vi "Vision Research Phantom Series PhInt PhInterpolateColorPAR.vi"(0 "Camera Number (1)":u32=1, 2 "CFA":T2 {"CFA" items=["CFA_NONE", "CFA_VRI", "CFA_VRIV6", "CFA_BAYER", "CFA_BAYERFLIP"]}, 3 "Algorithm":T1=1 items=["FAST_ALGORITHM"=1, "BEST_ALGORITHM"=5, "NO_DEMOSAICING"=6], 4 "pPixel In":u8[](array[numeric]), 5 "Error In (no error)":errorcluster, 7 "BITMAPINFOHEADER":T3) -> (14 "Camera Number out":u32=1, 16 "pPixel Out":u8[](array[numeric]), 19 "Error Out":errorcluster)   [LabVIEW 2013, in "VRI.lvlib"]
doc: "PhInt.dll\n\nPhInterpolateColorPAR\nPhInterpolateColorPAR(int Width, int Height, int BitCount, unsigned char * pPixel, int CFA, int Algorithm );\n\nParameters Description\nWidth Image width\nHeight Image height\nBitCount Bits per pixel\npPixel Pixel array pointer\nAlgorithm Interpolation algorithm code (BEST_ALGOTITHM, FAST_ALGORITHM)\nReturn Void\nComments A replacement for LabView of the PhMakeColor function\n\nWritten by:\nBLOOMY CONTROLS, INC\nWINDSOR, CT 06095, USA\n860-298-9925\nwww.bloomy.com\nV1.0.0\nMay, 2004"
uses:
  VRI.lvlib
  _Type Defs/BITMAPINFOHEADER.ctl
  _Type Defs/PhInt CFA.ctl
  _Type Defs/PhInt Algorithm.ctl
  Phantom DLLs/PhInt.dll
panel:
  # "For instructions on the use of this VI, press Ctrl+H to display the help window and move the mouse over the icon, controls, and indicators"
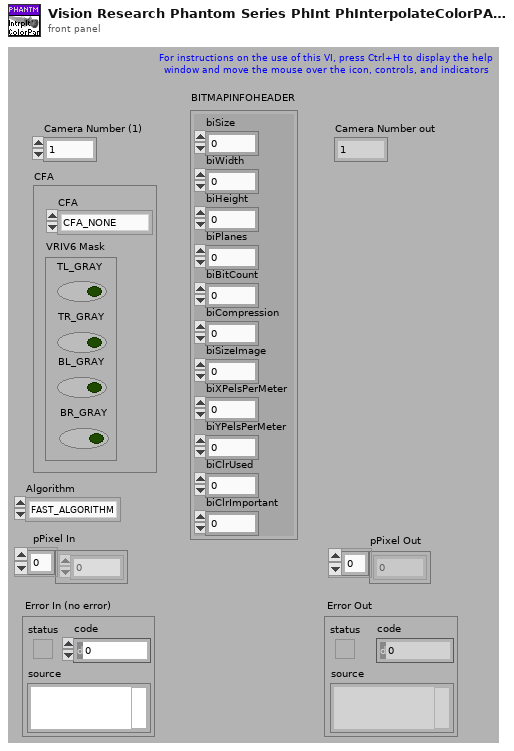
[diagram p1: front panel]
types:
  T1 = typedef "VRI.lvlib/PhInt Algorithm.ctl" = u32
  T2 = typedef "VRI.lvlib/PhInt CFA.ctl" = cluster{"CFA":u32, "VRIV6 Mask":cluster{"TL_GRAY":bool, "TR_GRAY":bool, "BL_GRAY":bool, "BR_GRAY":bool}}
  T3 = typedef "VRI.lvlib/BITMAPINFOHEADER.ctl" = cluster{"biSize":u32, "biWidth":i32, "biHeight":i32, "biPlanes":u16, "biBitCount":u16, "biCompression":u32, "biSizeImage":u32, "biXPelsPerMeter":i32, "biYPelsPerMeter":i32, "biClrUsed":u32, "biClrImportant":u32}
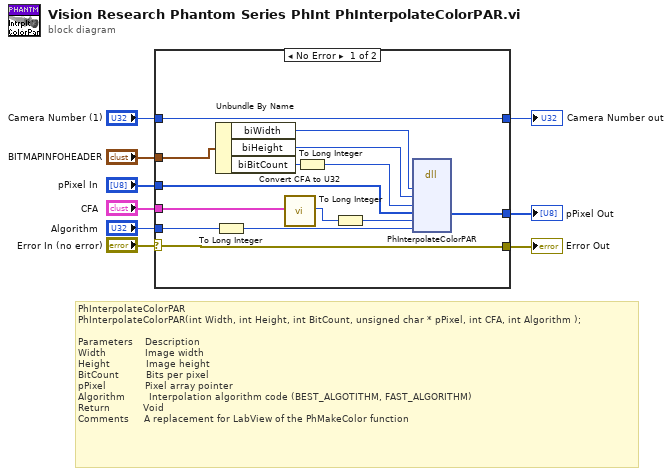
[diagram p0: block diagram]
diagram:
  # "PhInterpolateColorPAR\nPhInterpolateColorPAR(int Width, int Height, int BitCount, unsigned char * pPixel, int CFA, int Algorithm );\n\nParameters    Description\nWidth             Image width\nHeight            Image height\nBitCount         Bits per pixel\npPixel             Pixel array pointer\nAlgorithm        Interpolation algorithm code (BEST_ALGOTITHM, FAST_ALGORITHM)\nReturn           Void\nComments     A replacement for LabView of the PhMakeColor function"
  n1 = case shown="No Error" "Error In (no error)" {
    selector: "Error In (no error)" -> [w23 w25]
    tunnel: [w23 w25] -> w8
    tunnel: "Camera Number (1)" -> [w22 w24]
    tunnel: [w22 w24] -> w6
    tunnel: "BITMAPINFOHEADER" -> [w21 _]
    tunnel: "CFA" -> [w20 _]
    tunnel: "Algorithm" -> [w19 _]
    tunnel: [w18 _] -> w3
    tunnel: "pPixel In" -> [w17 _]
    frame No Error {
      n2 = Unbundle By Name(w21) -> ("biWidth"=w16:i32, "biHeight"=w15:i32, "biBitCount"=w14:u16)
      n3 = To Long Integer(number=w19) -> (32bit integer=w13:i32)
      n4 = call "Convert CFA to U32.vi"("CFA in"=w20) -> ("CFA out"=w11:u32)  [unwired: 18 out]
      n5 = To Long Integer(number=w14) -> (32bit integer=w12:i32)
      n6 = To Long Integer(number=w11) -> (32bit integer=w10:i32)
      n7 = dll-call lib="C:/Projects/SDK/32-bit/Vision Research Phantom Series Labview Driver/Phantom DLLs/PhInt.dll" fn="PhInterpolateColorPAR"("Width"=w16, "Height"=w15, "BitCount"=w12, "pPixel"=w17, "CFA"=w10, "Algorithm"=w13) -> ("pPixel"=w18:u8[])  [unwired: 8 in, 3 out]
    }
    frame Error {
    }
  }
  "Error Out" <- w8
  "Camera Number out" <- w6
  "pPixel Out" <- w3
